vi "Write Client List.vi"(8 "error in":errorcluster, 10 "Client List":T1[](array[typedef]), 11 "Client Manager in":refnum<class "Client Manager.lvclass">) -> (0 "error out":errorcluster, 3 "Client Manager out":refnum<class "Client Manager.lvclass">)   [LabVIEW 2014, in "Client Manager.lvclass"]
uses:
  Client Manager.lvclass
  Controls/Client Ref.ctl
  Client Manager.lvclass/Client Manager.ctl
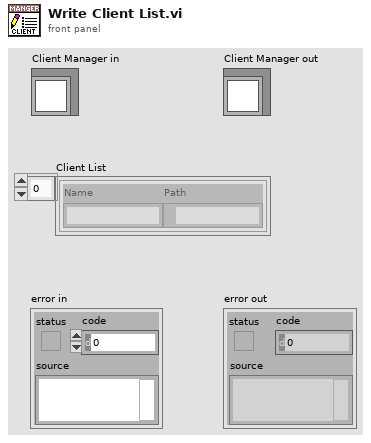
[diagram p1: front panel]
types:
  T1 = typedef "Client Ref.ctl" = cluster{"Name":string, "Path":path}
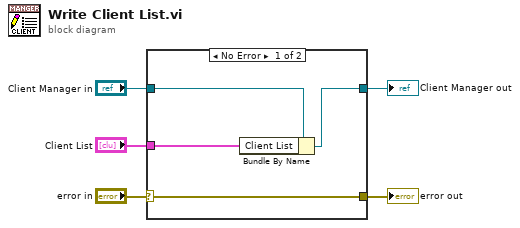
[diagram p0: block diagram]
diagram:
  n1 = case shown="No Error" "error in" {
    selector: "error in" -> [w9 w10]
    tunnel: [w9 w10] -> w4
    tunnel: [w7 w11] -> w2
    tunnel: "Client Manager in" -> [w8 w11]
    tunnel: "Client List" -> [w6 _]
    frame No Error {
      n2 = Bundle By Name(cluster=w8, "Client List"=w6) -> (w7:refnum<class "Client Manager.lvclass">)
    }
    frame Error {
    }
  }
  "error out" <- w4
  "Client Manager out" <- w2
